vi "ErrorEncoder.vi"(8 "Error In":errorcluster) -> (0 "Error Out":errorcluster)   [LabVIEW 2013]
uses:
  My Computer/Controls/ErrorHandlingClasses.ctl
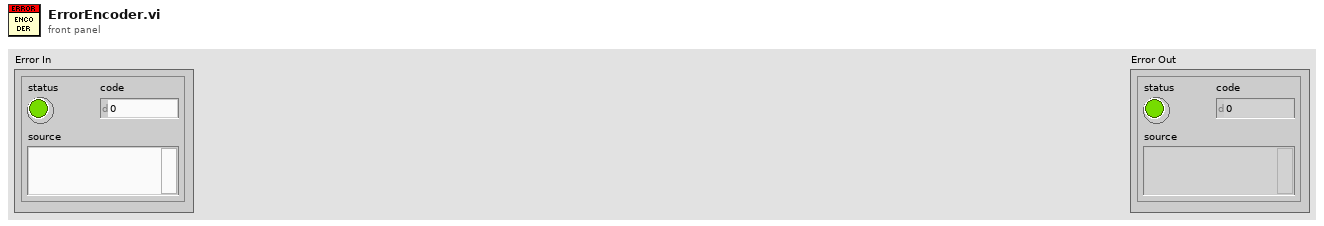
[diagram p1: front panel]
types:
  T1 = typedef "ErrorHandlingClasses.ctl" = enum16{"No Error", "Warning", "Error", "Critical Error"}
  T2 = enum16{"No Error", "1", "2", "3", "4", "5", "6", "7", "8", "9"}
  T3 = cluster{"Code":bool, "Priority":bool, "Class":bool}
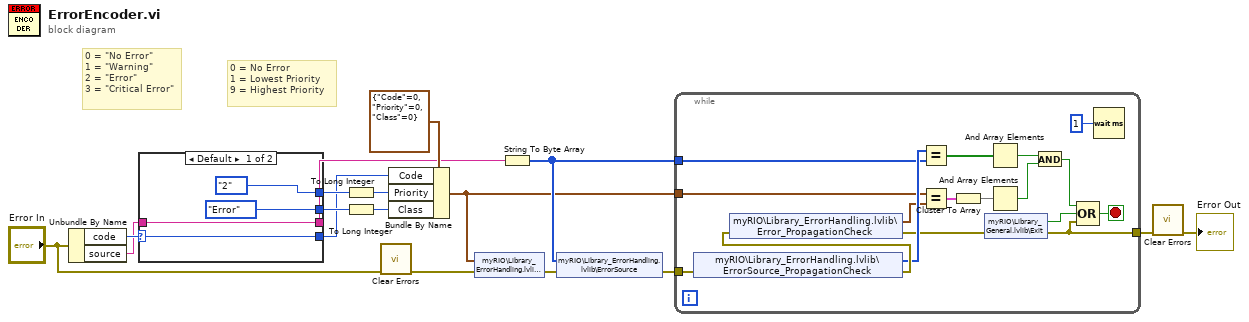
[diagram p0: block diagram]
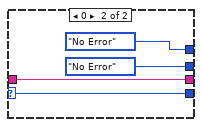
[diagram p2: hidden frame]
diagram:
  # "0 = No Error\n1 = Lowest Priority\n9 = Highest Priority"
  # "0 = \"No Error\"\n1 = \"Warning\"\n2 = \"Error\"\n3 = \"Critical Error\""
  n1 = Unbundle By Name("Error In") -> ("code"=w16:i32, "source"=w15:string)
  n2 = case shown="Default" w16 {
    selector: w16 -> [w21 w25]
    tunnel: [w21 w25] -> w10
    tunnel: w15 -> [w20 w24]
    tunnel: [w20 w24] -> w9
    tunnel: [ErrorHandlingClasses."Error" ErrorHandlingClasses."No Error"] -> w12
    tunnel: [T2."2" T2."No Error"] -> w14
    frame Default {
    }
    frame 0 {
    }
  }
  n3 = To Long Integer(number=w14) -> (32bit integer=w13:i32)
  n4 = To Long Integer(number=w12) -> (32bit integer=w11:i32)
  n5 = call <vilib>:"Clear Errors.vi"("error in (no error)"="Error In") -> ("error out"=w8:errorcluster)  [unwired: 6 in]
  n6 = Bundle By Name(cluster=cluster{"Code":i32, "Priority":i32, "Class":i32} {"Code"=0, "Priority"=0, "Class"=0} ("Error"), "Code"=w10, "Priority"=w13, "Class"=w11) -> (w4:cluster{"Code":i32, "Priority":i32, "Class":i32})
  n7 = shared-variable "myRIO\\Library_ErrorHandling.lvlib\\Error"(w4, error in=w8) -> (error out=w7:errorcluster)
  n8 = String To Byte Array(string=w9) -> (unsigned byte array=w5:u8[])
  n9 = shared-variable "myRIO\\Library_ErrorHandling.lvlib\\ErrorSource"(w5, error in=w7) -> (error out=w6:errorcluster)
  n10 = while {
    tunnel: w6 -> [w42]
    tunnel: [w26] -> w2
    tunnel: w5 -> [w38]
    tunnel: w4 -> [w32]
    stop <- w28 stop-if-true
    n11 = shared-variable "myRIO\\Library_ErrorHandling.lvlib\\ErrorSource_PropagationCheck"(error in=w42) -> (w39:u8[], error out=w41:errorcluster)
    n12 = shared-variable "myRIO\\Library_ErrorHandling.lvlib\\Error_PropagationCheck"(error in=w41) -> (w31:cluster{"Code":i32, "Priority":i32, "Class":i32}, error out=w30:errorcluster)
    n13 = Equal?(x=w39, y=w38) -> (x = y?=w37:bool[])
    n14 = Equal?(x=w32, y=w31) -> (x = y?=w35:T3)
    n15 = Cluster To Array(cluster=w35) -> (array=w34:bool[])
    n16 = shared-variable "myRIO\\Library_General.lvlib\\Exit"(error in=w30) -> (w27:bool, error out=w26:errorcluster)
    n17 = And Array Elements(Boolean array=w37) -> (logical AND=w36:bool)
    n18 = And Array Elements(Boolean array=w34) -> (logical AND=w33:bool)
    n19 = And(x=w36, y=w33) -> (x .and. y?=w29:bool)
    n20 = Compound Arithmetic op=OR(w29, w27, w26) -> (w28:bool)
    n21 = Wait (ms)(milliseconds to wait=u32 1) -> ()  [unwired: 1 out]
  }
  n22 = call <vilib>:"Clear Errors.vi"("error in (no error)"=w2) -> ("error out"=→"Error Out":errorcluster)  [unwired: 6 in]
